vi "data_2.vi"() -> ()   [LabVIEW 2020]
panel:
  in  "ROI Coordinates":T1={"XYZ Start"=[{"X"=-1.0, "Y"=-1.0, "Z"=0.0}, {"X"=-1.0, "Y"=-0.99, "Z"=0.0}, {"X"=-1.0, "Y"=-0.98, "Z"=0.0}, {"X"=-1.0, "Y"=-0.97, "Z"=0.0}, {"X"=-1.0, "Y"=-0.96, "Z"=0.0}, {"X"=-1.0, "Y"=-0.95, "Z"=0.0}, {"X"=-1.0, "Y"=-0.94, "Z"=0.0}, {"X"=-1.0, "Y"=-0.93, "Z"=0.0}, {"X"=-1.0, "Y"=-0.92, "Z"=0.0}, {"X"=-1.0, "Y"=-0.91, "Z"=0.0}, {"X"=-1.0, "Y"=-0.9, "Z"=0.0}, {"X"=-1.0, "Y"=-0.89, "Z"=0.0}, {"X"=-1.0, "Y"=-0.88, "Z"=0.0}, {"X"=-1.0, "Y"=-0.87, "Z"=0.0}, {"X"=-1.0, "Y"=-0.86, "Z"=0.0}, {"X"=-1.0, "Y"=-0.85, "Z"=0.0}, {"X"=-1.0, "Y"=-0.84, "Z"=0.0}, {"X"=-1.0, "Y"=-0.83, "Z"=0.0}, {"X"=-1.0, "Y"=-0.82, "Z"=0.0}, {"X"=-1.0, "Y"=-0.81, "Z"=0.0}, {"X"=-1.0, "Y"=-0.8, "Z"=0.0}, {"X"=-1.0, "Y"=-0.79, "Z"=0.0}, {"X"=-1.0, "Y"=-0.78, "Z"=0.0}, {"X"=-1.0, "Y"=-0.77, "Z"=0.0}, {"X"=-1.0, "Y"=-0.76, "Z"=0.0}, {"X"=-1.0, "Y"=-0.75, "Z"=0.0}, {"X"=-1.0, "Y"=-0.74, "Z"=0.0}, {"X"=-1.0, "Y"=-0.73, "Z"=0.0}, {"X"=-1.0, "Y"=-0.72, "Z"=0.0}, {"X"=-1.0, "Y"=-0.71, "Z"=0.0}, {"X"=-1.0, "Y"=-0.7, "Z"=0.0}, {"X"=-1.0, "Y"=-0.69, "Z"=0.0}, {"X"=-1.0, "Y"=-0.68, "Z"=0.0}, {"X"=-1.0, "Y"=-0.67, "Z"=0.0}, {"X"=-1.0, "Y"=-0.66, "Z"=0.0}, {"X"=-1.0, "Y"=-0.65, "Z"=0.0}, {"X"=-1.0, "Y"=-0.64, "Z"=0.0}, {"X"=-1.0, "Y"=-0.63, "Z"=0.0}, {"X"=-1.0, "Y"=-0.62, "Z"=0.0}, {"X"=-1.0, "Y"=-0.61, "Z"=0.0}, {"X"=-1.0, "Y"=-0.6, "Z"=0.0}, {"X"=-1.0, "Y"=-0.59, "Z"=0.0}, {"X"=-1.0, "Y"=-0.58, "Z"=0.0}, {"X"=-1.0, "Y"=-0.57, "Z"=0.0}, {"X"=-1.0, "Y"=-0.56, "Z"=0.0}, {"X"=-1.0, "Y"=-0.55, "Z"=0.0}, {"X"=-1.0, "Y"=-0.54, "Z"=0.0}, {"X"=-1.0, "Y"=-0.53, "Z"=0.0}, {"X"=-1.0, "Y"=-0.52, "Z"=0.0}, {"X"=-1.0, "Y"=-0.51, "Z"=0.0}, {"X"=-1.0, "Y"=-0.5, "Z"=0.0}, {"X"=-1.0, "Y"=-0.49, "Z"=0.0}, {"X"=-1.0, "Y"=-0.48, "Z"=0.0}, {"X"=-1.0, "Y"=-0.47, "Z"=0.0}, {"X"=-1.0, "Y"=-0.46, "Z"=0.0}, {"X"=-1.0, "Y"=-0.45, "Z"=0.0}, {"X"=-1.0, "Y"=-0.44, "Z"=0.0}, {"X"=-1.0, "Y"=-0.43, "Z"=0.0}, {"X"=-1.0, "Y"=-0.42, "Z"=0.0}, {"X"=-1.0, "Y"=-0.41, "Z"=0.0}, {"X"=-1.0, "Y"=-0.4, "Z"=0.0}, {"X"=-1.0, "Y"=-0.39, "Z"=0.0}, {"X"=-1.0, "Y"=-0.38, "Z"=0.0}, {"X"=-1.0, "Y"=-0.37, "Z"=0.0}, {"X"=-1.0, "Y"=-0.36, "Z"=0.0}, {"X"=-1.0, "Y"=-0.35, "Z"=0.0}, {"X"=-1.0, "Y"=-0.34, "Z"=0.0}, {"X"=-1.0, "Y"=-0.33, "Z"=0.0}, {"X"=-1.0, "Y"=-0.32, "Z"=0.0}, {"X"=-1.0, "Y"=-0.31, "Z"=0.0}, {"X"=-1.0, "Y"=-0.3, "Z"=0.0}, {"X"=-1.0, "Y"=-0.29, "Z"=0.0}, {"X"=-1.0, "Y"=-0.28, "Z"=0.0}, {"X"=-1.0, "Y"=-0.27, "Z"=0.0}, {"X"=-1.0, "Y"=-0.26, "Z"=0.0}, {"X"=-1.0, "Y"=-0.25, "Z"=0.0}, {"X"=-1.0, "Y"=-0.24, "Z"=0.0}, {"X"=-1.0, "Y"=-0.23, "Z"=0.0}, {"X"=-1.0, "Y"=-0.22, "Z"=0.0}, {"X"=-1.0, "Y"=-0.21, "Z"=0.0}, {"X"=-1.0, "Y"=-0.2, "Z"=0.0}, {"X"=-1.0, "Y"=-0.19, "Z"=0.0}, {"X"=-1.0, "Y"=-0.18, "Z"=0.0}, {"X"=-1.0, "Y"=-0.17, "Z"=0.0}, {"X"=-1.0, "Y"=-0.16, "Z"=0.0}, {"X"=-1.0, "Y"=-0.15, "Z"=0.0}, {"X"=-1.0, "Y"=-0.14, "Z"=0.0}, {"X"=-1.0, "Y"=-0.13, "Z"=0.0}, {"X"=-1.0, "Y"=-0.12, "Z"=0.0}, {"X"=-1.0, "Y"=-0.11, "Z"=0.0}, {"X"=-1.0, "Y"=-0.1, "Z"=0.0}, {"X"=-1.0, "Y"=-0.09, "Z"=0.0}, {"X"=-1.0, "Y"=-0.08, "Z"=0.0}, {"X"=-1.0, "Y"=-0.07, "Z"=0.0}, {"X"=-1.0, "Y"=-0.06, "Z"=0.0}, {"X"=-1.0, "Y"=-0.05, "Z"=0.0}, {"X"=-1.0, "Y"=-0.04, "Z"=0.0}, {"X"=-1.0, "Y"=-0.03, "Z"=0.0}, {"X"=-1.0, "Y"=-0.02, "Z"=0.0}, {"X"=-1.0, "Y"=-0.01, "Z"=0.0}, {"X"=-1.0, "Y"=0.0, "Z"=0.0}, {"X"=-1.0, "Y"=0.01, "Z"=0.0}, {"X"=-1.0, "Y"=0.02, "Z"=0.0}, {"X"=-1.0, "Y"=0.03, "Z"=0.0}, {"X"=-1.0, "Y"=0.04, "Z"=0.0}, {"X"=-1.0, "Y"=0.05, "Z"=0.0}, {"X"=-1.0, "Y"=0.06, "Z"=0.0}, {"X"=-1.0, "Y"=0.07, "Z"=0.0}, {"X"=-1.0, "Y"=0.08, "Z"=0.0}, {"X"=-1.0, "Y"=0.09, "Z"=0.0}, {"X"=-1.0, "Y"=0.1, "Z"=0.0}, {"X"=-1.0, "Y"=0.11, "Z"=0.0}, {"X"=-1.0, "Y"=0.12, "Z"=0.0}, {"X"=-1.0, "Y"=0.13, "Z"=0.0}, {"X"=-1.0, "Y"=0.14, "Z"=0.0}, {"X"=-1.0, "Y"=0.15, "Z"=0.0}, {"X"=-1.0, "Y"=0.16, "Z"=0.0}, {"X"=-1.0, "Y"=0.17, "Z"=0.0}, {"X"=-1.0, "Y"=0.18, "Z"=0.0}, {"X"=-1.0, "Y"=0.19, "Z"=0.0}, {"X"=-1.0, "Y"=0.2, "Z"=0.0}, {"X"=-1.0, "Y"=0.21, "Z"=0.0}, {"X"=-1.0, "Y"=0.22, "Z"=0.0}, {"X"=-1.0, "Y"=0.23, "Z"=0.0}, {"X"=-1.0, "Y"=0.24, "Z"=0.0}, {"X"=-1.0, "Y"=0.25, "Z"=0.0}, {"X"=-1.0, "Y"=0.26, "Z"=0.0}, {"X"=-1.0, "Y"=0.27, "Z"=0.0}, {"X"=-1.0, "Y"=0.28, "Z"=0.0}, {"X"=-1.0, "Y"=0.29, "Z"=0.0}, {"X"=-1.0, "Y"=0.3, "Z"=0.0}, {"X"=-1.0, "Y"=0.31, "Z"=0.0}, {"X"=-1.0, "Y"=0.32, "Z"=0.0}, {"X"=-1.0, "Y"=0.33, "Z"=0.0}, {"X"=-1.0, "Y"=0.34, "Z"=0.0}, {"X"=-1.0, "Y"=0.35, "Z"=0.0}, {"X"=-1.0, "Y"=0.36, "Z"=0.0}, {"X"=-1.0, "Y"=0.37, "Z"=0.0}, {"X"=-1.0, "Y"=0.38, "Z"=0.0}, {"X"=-1.0, "Y"=0.39, "Z"=0.0}, {"X"=-1.0, "Y"=0.4, "Z"=0.0}, {"X"=-1.0, "Y"=0.41, "Z"=0.0}, {"X"=-1.0, "Y"=0.42, "Z"=0.0}, {"X"=-1.0, "Y"=0.43, "Z"=0.0}, {"X"=-1.0, "Y"=0.44, "Z"=0.0}, {"X"=-1.0, "Y"=0.45, "Z"=0.0}, {"X"=-1.0, "Y"=0.46, "Z"=0.0}, {"X"=-1.0, "Y"=0.47, "Z"=0.0}, {"X"=-1.0, "Y"=0.48, "Z"=0.0}, {"X"=-1.0, "Y"=0.49, "Z"=0.0}, {"X"=-1.0, "Y"=0.5, "Z"=0.0}, {"X"=-1.0, "Y"=0.51, "Z"=0.0}, {"X"=-1.0, "Y"=0.52, "Z"=0.0}, {"X"=-1.0, "Y"=0.53, "Z"=0.0}, {"X"=-1.0, "Y"=0.54, "Z"=0.0}, {"X"=-1.0, "Y"=0.55, "Z"=0.0}, {"X"=-1.0, "Y"=0.56, "Z"=0.0}, {"X"=-1.0, "Y"=0.57, "Z"=0.0}, {"X"=-1.0, "Y"=0.58, "Z"=0.0}, {"X"=-1.0, "Y"=0.59, "Z"=0.0}, {"X"=-1.0, "Y"=0.6, "Z"=0.0}, {"X"=-1.0, "Y"=0.61, "Z"=0.0}, {"X"=-1.0, "Y"=0.62, "Z"=0.0}, {"X"=-1.0, "Y"=0.63, "Z"=0.0}, {"X"=-1.0, "Y"=0.64, "Z"=0.0}, {"X"=-1.0, "Y"=0.65, "Z"=0.0}, {"X"=-1.0, "Y"=0.66, "Z"=0.0}, {"X"=-1.0, "Y"=0.67, "Z"=0.0}, {"X"=-1.0, "Y"=0.68, "Z"=0.0}, {"X"=-1.0, "Y"=0.69, "Z"=0.0}, {"X"=-1.0, "Y"=0.7, "Z"=0.0}, {"X"=-1.0, "Y"=0.71, "Z"=0.0}, {"X"=-1.0, "Y"=0.72, "Z"=0.0}, {"X"=-1.0, "Y"=0.73, "Z"=0.0}, {"X"=-1.0, "Y"=0.74, "Z"=0.0}, {"X"=-1.0, "Y"=0.75, "Z"=0.0}, {"X"=-1.0, "Y"=0.76, "Z"=0.0}, {"X"=-1.0, "Y"=0.77, "Z"=0.0}, {"X"=-1.0, "Y"=0.78, "Z"=0.0}, {"X"=-1.0, "Y"=0.79, "Z"=0.0}, {"X"=-1.0, "Y"=0.8, "Z"=0.0}, {"X"=-1.0, "Y"=0.81, "Z"=0.0}, {"X"=-1.0, "Y"=0.82, "Z"=0.0}, {"X"=-1.0, "Y"=0.83, "Z"=0.0}, {"X"=-1.0, "Y"=0.84, "Z"=0.0}, {"X"=-1.0, "Y"=0.85, "Z"=0.0}, {"X"=-1.0, "Y"=0.86, "Z"=0.0}, {"X"=-1.0, "Y"=0.87, "Z"=0.0}, {"X"=-1.0, "Y"=0.88, "Z"=0.0}, {"X"=-1.0, "Y"=0.89, "Z"=0.0}, {"X"=-1.0, "Y"=0.9, "Z"=0.0}, {"X"=-1.0, "Y"=0.91, "Z"=0.0}, {"X"=-1.0, "Y"=0.92, "Z"=0.0}, {"X"=-1.0, "Y"=0.93, "Z"=0.0}, {"X"=-1.0, "Y"=0.94, "Z"=0.0}, {"X"=-1.0, "Y"=0.95, "Z"=0.0}, {"X"=-1.0, "Y"=0.96, "Z"=0.0}, {"X"=-1.0, "Y"=0.97, "Z"=0.0}, {"X"=-1.0, "Y"=0.98, "Z"=0.0}, {"X"=-1.0, "Y"=0.99, "Z"=0.0}], "XYZ Stop"=[{"X"=1.0, "Y"=-1.0, "Z"=0.0}, {"X"=1.0, "Y"=-0.99, "Z"=0.0}, {"X"=1.0, "Y"=-0.98, "Z"=0.0}, {"X"=1.0, "Y"=-0.97, "Z"=0.0}, {"X"=1.0, "Y"=-0.96, "Z"=0.0}, {"X"=1.0, "Y"=-0.95, "Z"=0.0}, {"X"=1.0, "Y"=-0.94, "Z"=0.0}, {"X"=1.0, "Y"=-0.93, "Z"=0.0}, {"X"=1.0, "Y"=-0.92, "Z"=0.0}, {"X"=1.0, "Y"=-0.91, "Z"=0.0}, {"X"=1.0, "Y"=-0.9, "Z"=0.0}, {"X"=1.0, "Y"=-0.89, "Z"=0.0}, {"X"=1.0, "Y"=-0.88, "Z"=0.0}, {"X"=1.0, "Y"=-0.87, "Z"=0.0}, {"X"=1.0, "Y"=-0.86, "Z"=0.0}, {"X"=1.0, "Y"=-0.85, "Z"=0.0}, {"X"=1.0, "Y"=-0.84, "Z"=0.0}, {"X"=1.0, "Y"=-0.83, "Z"=0.0}, {"X"=1.0, "Y"=-0.82, "Z"=0.0}, {"X"=1.0, "Y"=-0.81, "Z"=0.0}, {"X"=1.0, "Y"=-0.8, "Z"=0.0}, {"X"=1.0, "Y"=-0.79, "Z"=0.0}, {"X"=1.0, "Y"=-0.78, "Z"=0.0}, {"X"=1.0, "Y"=-0.77, "Z"=0.0}, {"X"=1.0, "Y"=-0.76, "Z"=0.0}, {"X"=1.0, "Y"=-0.75, "Z"=0.0}, {"X"=1.0, "Y"=-0.74, "Z"=0.0}, {"X"=1.0, "Y"=-0.73, "Z"=0.0}, {"X"=1.0, "Y"=-0.72, "Z"=0.0}, {"X"=1.0, "Y"=-0.71, "Z"=0.0}, {"X"=1.0, "Y"=-0.7, "Z"=0.0}, {"X"=1.0, "Y"=-0.69, "Z"=0.0}, {"X"=1.0, "Y"=-0.68, "Z"=0.0}, {"X"=1.0, "Y"=-0.67, "Z"=0.0}, {"X"=1.0, "Y"=-0.66, "Z"=0.0}, {"X"=1.0, "Y"=-0.65, "Z"=0.0}, {"X"=1.0, "Y"=-0.64, "Z"=0.0}, {"X"=1.0, "Y"=-0.63, "Z"=0.0}, {"X"=1.0, "Y"=-0.62, "Z"=0.0}, {"X"=1.0, "Y"=-0.61, "Z"=0.0}, {"X"=1.0, "Y"=-0.6, "Z"=0.0}, {"X"=1.0, "Y"=-0.59, "Z"=0.0}, {"X"=1.0, "Y"=-0.58, "Z"=0.0}, {"X"=1.0, "Y"=-0.57, "Z"=0.0}, {"X"=1.0, "Y"=-0.56, "Z"=0.0}, {"X"=1.0, "Y"=-0.55, "Z"=0.0}, {"X"=1.0, "Y"=-0.54, "Z"=0.0}, {"X"=1.0, "Y"=-0.53, "Z"=0.0}, {"X"=1.0, "Y"=-0.52, "Z"=0.0}, {"X"=1.0, "Y"=-0.51, "Z"=0.0}, {"X"=1.0, "Y"=-0.5, "Z"=0.0}, {"X"=1.0, "Y"=-0.49, "Z"=0.0}, {"X"=1.0, "Y"=-0.48, "Z"=0.0}, {"X"=1.0, "Y"=-0.47, "Z"=0.0}, {"X"=1.0, "Y"=-0.46, "Z"=0.0}, {"X"=1.0, "Y"=-0.45, "Z"=0.0}, {"X"=1.0, "Y"=-0.44, "Z"=0.0}, {"X"=1.0, "Y"=-0.43, "Z"=0.0}, {"X"=1.0, "Y"=-0.42, "Z"=0.0}, {"X"=1.0, "Y"=-0.41, "Z"=0.0}, {"X"=1.0, "Y"=-0.4, "Z"=0.0}, {"X"=1.0, "Y"=-0.39, "Z"=0.0}, {"X"=1.0, "Y"=-0.38, "Z"=0.0}, {"X"=1.0, "Y"=-0.37, "Z"=0.0}, {"X"=1.0, "Y"=-0.36, "Z"=0.0}, {"X"=1.0, "Y"=-0.35, "Z"=0.0}, {"X"=1.0, "Y"=-0.34, "Z"=0.0}, {"X"=1.0, "Y"=-0.33, "Z"=0.0}, {"X"=1.0, "Y"=-0.32, "Z"=0.0}, {"X"=1.0, "Y"=-0.31, "Z"=0.0}, {"X"=1.0, "Y"=-0.3, "Z"=0.0}, {"X"=1.0, "Y"=-0.29, "Z"=0.0}, {"X"=1.0, "Y"=-0.28, "Z"=0.0}, {"X"=1.0, "Y"=-0.27, "Z"=0.0}, {"X"=1.0, "Y"=-0.26, "Z"=0.0}, {"X"=1.0, "Y"=-0.25, "Z"=0.0}, {"X"=1.0, "Y"=-0.24, "Z"=0.0}, {"X"=1.0, "Y"=-0.23, "Z"=0.0}, {"X"=1.0, "Y"=-0.22, "Z"=0.0}, {"X"=1.0, "Y"=-0.21, "Z"=0.0}, {"X"=1.0, "Y"=-0.2, "Z"=0.0}, {"X"=1.0, "Y"=-0.19, "Z"=0.0}, {"X"=1.0, "Y"=-0.18, "Z"=0.0}, {"X"=1.0, "Y"=-0.17, "Z"=0.0}, {"X"=1.0, "Y"=-0.16, "Z"=0.0}, {"X"=1.0, "Y"=-0.15, "Z"=0.0}, {"X"=1.0, "Y"=-0.14, "Z"=0.0}, {"X"=1.0, "Y"=-0.13, "Z"=0.0}, {"X"=1.0, "Y"=-0.12, "Z"=0.0}, {"X"=1.0, "Y"=-0.11, "Z"=0.0}, {"X"=1.0, "Y"=-0.1, "Z"=0.0}, {"X"=1.0, "Y"=-0.09, "Z"=0.0}, {"X"=1.0, "Y"=-0.08, "Z"=0.0}, {"X"=1.0, "Y"=-0.07, "Z"=0.0}, {"X"=1.0, "Y"=-0.06, "Z"=0.0}, {"X"=1.0, "Y"=-0.05, "Z"=0.0}, {"X"=1.0, "Y"=-0.04, "Z"=0.0}, {"X"=1.0, "Y"=-0.03, "Z"=0.0}, {"X"=1.0, "Y"=-0.02, "Z"=0.0}, {"X"=1.0, "Y"=-0.01, "Z"=0.0}, {"X"=1.0, "Y"=0.0, "Z"=0.0}, {"X"=1.0, "Y"=0.01, "Z"=0.0}, {"X"=1.0, "Y"=0.02, "Z"=0.0}, {"X"=1.0, "Y"=0.03, "Z"=0.0}, {"X"=1.0, "Y"=0.04, "Z"=0.0}, {"X"=1.0, "Y"=0.05, "Z"=0.0}, {"X"=1.0, "Y"=0.06, "Z"=0.0}, {"X"=1.0, "Y"=0.07, "Z"=0.0}, {"X"=1.0, "Y"=0.08, "Z"=0.0}, {"X"=1.0, "Y"=0.09, "Z"=0.0}, {"X"=1.0, "Y"=0.1, "Z"=0.0}, {"X"=1.0, "Y"=0.11, "Z"=0.0}, {"X"=1.0, "Y"=0.12, "Z"=0.0}, {"X"=1.0, "Y"=0.13, "Z"=0.0}, {"X"=1.0, "Y"=0.14, "Z"=0.0}, {"X"=1.0, "Y"=0.15, "Z"=0.0}, {"X"=1.0, "Y"=0.16, "Z"=0.0}, {"X"=1.0, "Y"=0.17, "Z"=0.0}, {"X"=1.0, "Y"=0.18, "Z"=0.0}, {"X"=1.0, "Y"=0.19, "Z"=0.0}, {"X"=1.0, "Y"=0.2, "Z"=0.0}, {"X"=1.0, "Y"=0.21, "Z"=0.0}, {"X"=1.0, "Y"=0.22, "Z"=0.0}, {"X"=1.0, "Y"=0.23, "Z"=0.0}, {"X"=1.0, "Y"=0.24, "Z"=0.0}, {"X"=1.0, "Y"=0.25, "Z"=0.0}, {"X"=1.0, "Y"=0.26, "Z"=0.0}, {"X"=1.0, "Y"=0.27, "Z"=0.0}, {"X"=1.0, "Y"=0.28, "Z"=0.0}, {"X"=1.0, "Y"=0.29, "Z"=0.0}, {"X"=1.0, "Y"=0.3, "Z"=0.0}, {"X"=1.0, "Y"=0.31, "Z"=0.0}, {"X"=1.0, "Y"=0.32, "Z"=0.0}, {"X"=1.0, "Y"=0.33, "Z"=0.0}, {"X"=1.0, "Y"=0.34, "Z"=0.0}, {"X"=1.0, "Y"=0.35, "Z"=0.0}, {"X"=1.0, "Y"=0.36, "Z"=0.0}, {"X"=1.0, "Y"=0.37, "Z"=0.0}, {"X"=1.0, "Y"=0.38, "Z"=0.0}, {"X"=1.0, "Y"=0.39, "Z"=0.0}, {"X"=1.0, "Y"=0.4, "Z"=0.0}, {"X"=1.0, "Y"=0.41, "Z"=0.0}, {"X"=1.0, "Y"=0.42, "Z"=0.0}, {"X"=1.0, "Y"=0.43, "Z"=0.0}, {"X"=1.0, "Y"=0.44, "Z"=0.0}, {"X"=1.0, "Y"=0.45, "Z"=0.0}, {"X"=1.0, "Y"=0.46, "Z"=0.0}, {"X"=1.0, "Y"=0.47, "Z"=0.0}, {"X"=1.0, "Y"=0.48, "Z"=0.0}, {"X"=1.0, "Y"=0.49, "Z"=0.0}, {"X"=1.0, "Y"=0.5, "Z"=0.0}, {"X"=1.0, "Y"=0.51, "Z"=0.0}, {"X"=1.0, "Y"=0.52, "Z"=0.0}, {"X"=1.0, "Y"=0.53, "Z"=0.0}, {"X"=1.0, "Y"=0.54, "Z"=0.0}, {"X"=1.0, "Y"=0.55, "Z"=0.0}, {"X"=1.0, "Y"=0.56, "Z"=0.0}, {"X"=1.0, "Y"=0.57, "Z"=0.0}, {"X"=1.0, "Y"=0.58, "Z"=0.0}, {"X"=1.0, "Y"=0.59, "Z"=0.0}, {"X"=1.0, "Y"=0.6, "Z"=0.0}, {"X"=1.0, "Y"=0.61, "Z"=0.0}, {"X"=1.0, "Y"=0.62, "Z"=0.0}, {"X"=1.0, "Y"=0.63, "Z"=0.0}, {"X"=1.0, "Y"=0.64, "Z"=0.0}, {"X"=1.0, "Y"=0.65, "Z"=0.0}, {"X"=1.0, "Y"=0.66, "Z"=0.0}, {"X"=1.0, "Y"=0.67, "Z"=0.0}, {"X"=1.0, "Y"=0.68, "Z"=0.0}, {"X"=1.0, "Y"=0.69, "Z"=0.0}, {"X"=1.0, "Y"=0.7, "Z"=0.0}, {"X"=1.0, "Y"=0.71, "Z"=0.0}, {"X"=1.0, "Y"=0.72, "Z"=0.0}, {"X"=1.0, "Y"=0.73, "Z"=0.0}, {"X"=1.0, "Y"=0.74, "Z"=0.0}, {"X"=1.0, "Y"=0.75, "Z"=0.0}, {"X"=1.0, "Y"=0.76, "Z"=0.0}, {"X"=1.0, "Y"=0.77, "Z"=0.0}, {"X"=1.0, "Y"=0.78, "Z"=0.0}, {"X"=1.0, "Y"=0.79, "Z"=0.0}, {"X"=1.0, "Y"=0.8, "Z"=0.0}, {"X"=1.0, "Y"=0.81, "Z"=0.0}, {"X"=1.0, "Y"=0.82, "Z"=0.0}, {"X"=1.0, "Y"=0.83, "Z"=0.0}, {"X"=1.0, "Y"=0.84, "Z"=0.0}, {"X"=1.0, "Y"=0.85, "Z"=0.0}, {"X"=1.0, "Y"=0.86, "Z"=0.0}, {"X"=1.0, "Y"=0.87, "Z"=0.0}, {"X"=1.0, "Y"=0.88, "Z"=0.0}, {"X"=1.0, "Y"=0.89, "Z"=0.0}, {"X"=1.0, "Y"=0.9, "Z"=0.0}, {"X"=1.0, "Y"=0.91, "Z"=0.0}, {"X"=1.0, "Y"=0.92, "Z"=0.0}, {"X"=1.0, "Y"=0.93, "Z"=0.0}, {"X"=1.0, "Y"=0.94, "Z"=0.0}, {"X"=1.0, "Y"=0.95, "Z"=0.0}, {"X"=1.0, "Y"=0.96, "Z"=0.0}, {"X"=1.0, "Y"=0.97, "Z"=0.0}, {"X"=1.0, "Y"=0.98, "Z"=0.0}, {"X"=1.0, "Y"=0.99, "Z"=0.0}]}
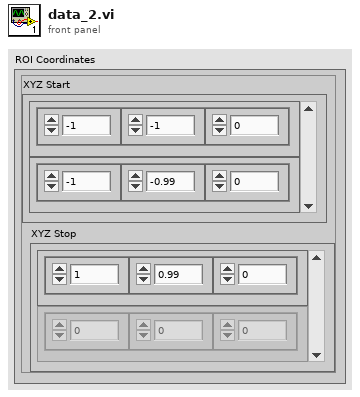
[diagram p1: front panel]
types:
  T1 = cluster{"XYZ Start":cluster{"X":sgl, "Y":sgl, "Z":sgl}[], "XYZ Stop":cluster{"X":sgl, "Y":sgl, "Z":sgl}[]}
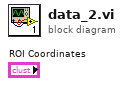
[diagram p0: block diagram]
diagram:
